vi "Write.vi"(8 "error in (no error)":errorcluster, 10 "Message":string, 11 "Serial in":refnum<class "Serial.lvclass">) -> (0 "error out":errorcluster, 3 "Serial out":refnum<class "Serial.lvclass">)   [LabVIEW 2021, in "Serial.lvclass"]
uses:
  Serial.lvclass
  Serial.lvclass/Serial.ctl
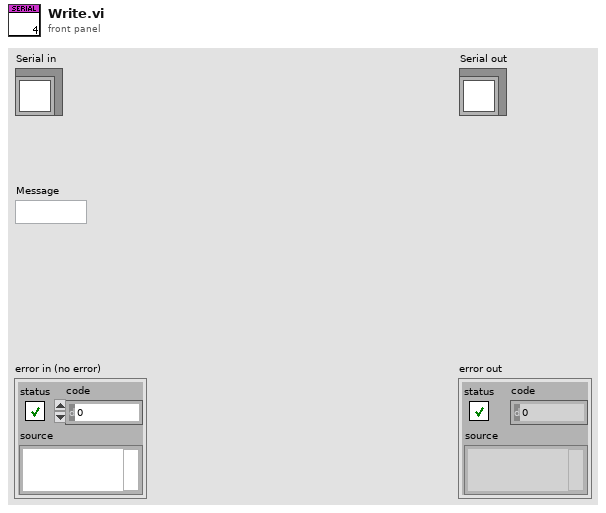
[diagram p1: front panel]
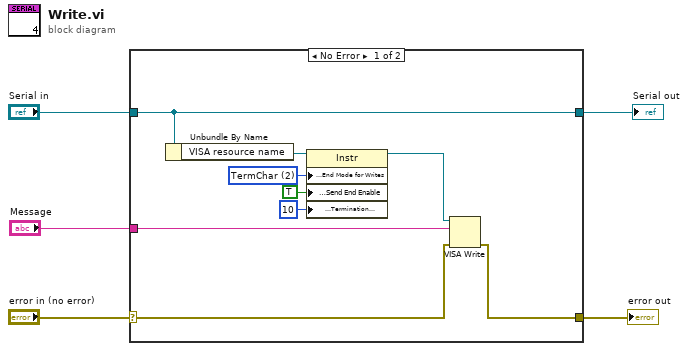
[diagram p0: block diagram]
diagram:
  n1 = case shown="No Error" "error in (no error)" {
    selector: "error in (no error)" -> [w11 w16]
    tunnel: [w12 w16] -> w4
    tunnel: "Serial in" -> [w14 w15]
    tunnel: [w14 w15] -> w2
    tunnel: "Message" -> [w13 _]
    frame No Error {
      w10 = u16 2 items=["None", "Last Bit", "TermChar", "Break"] ("Serial Settings:End Mode for Writes")
      n2 = Unbundle By Name(w14) -> ("VISA resource name"=w7:refnum<visa-resource-name>)
      n3 = property class="Instr"(reference=w7, "Serial Settings:End Mode for Writes"=w10, "Message Based Settings:Send End Enable"=TRUE, "Message Based Settings:Termination Character"=u8 10) -> (reference out=w6:refnum<visa-resource-name>)  [unwired: 1 in, 1 out]
      n4 = VISA Write(VISA resource name=w6, write buffer=w13, error in (no error)=w11) -> (error out=w12:errorcluster)  [unwired: 2 out]
    }
    frame Error {
    }
  }
  "error out" <- w4
  "Serial out" <- w2
